vi "Display.vi"(8 "error in":errorcluster, 11 "Input (String) in":refnum<class "Gif - Input (String).lvclass">) -> (0 "error out":errorcluster, 3 "Input (String) out":refnum<class "Gif - Input (String).lvclass">)   [LabVIEW 2020, in "Pop-Up.lvlib" / "Gif - Input (String).lvclass"]
doc: "This vi will display the input pop up waiting for a type string input from the user while displaying a custom graphic to the user.\n\n<b>Code Developed By:</b>\nDaniel Coons\nTechnology Service Corporation\n1983 S Liberty Drive\nBloomington, IN 47403\nPhone: 812 558-7100\ndaniel.coons@tsc.com\nwww.tsc.com/atcs"
uses:
  Gif - Input (String).lvclass
  C:/Development/tsc-pop-up/Popup/Popup.lvclass
  C:/Development/tsc-pop-up/Gif/Gif Parent.lvclass
  Gif - Input (String).lvclass/Gif - Input (String).ctl
  Popup/Popup.lvclass/Popup.ctl
  Gif Parent.lvclass/Gif Parent.ctl
  Popup/Data Member Access/Read Theme.vi
  Read Delays.vi
  Read Gif Images.vi
  Theme/Theme.lvclass
  Popup/Popup.lvclass
  user32.dll
panel:
  in  "closer":bool
  out "header":bool
  in  "OK":bool
  in  "Input":string
  out "Input value out":string
  out "2D Picture":picture
  out "Message":string
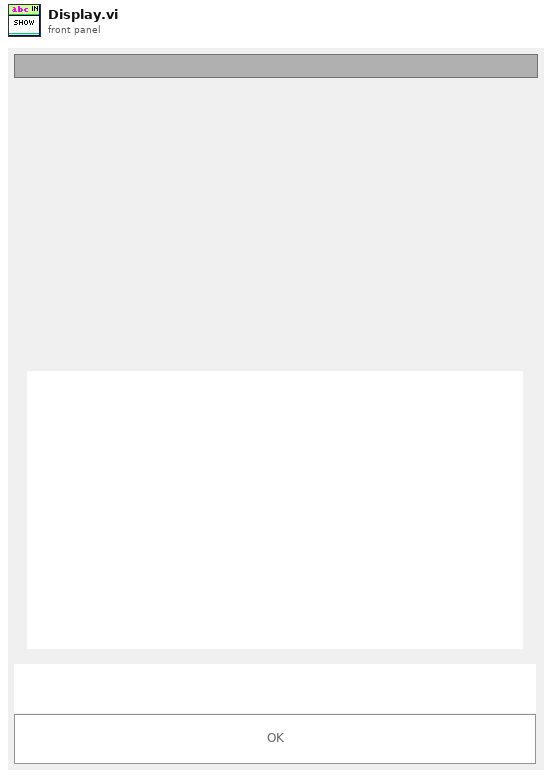
[diagram p1: front panel]
types:
  T1 = typedef "LVPoint32TypeDef.ctl" = cluster{"Horizontal":i32, "Vertical":i32}
  T2 = typedef "LVPositionTypeDef.ctl" = cluster{"Left":i32, "Top":i32}
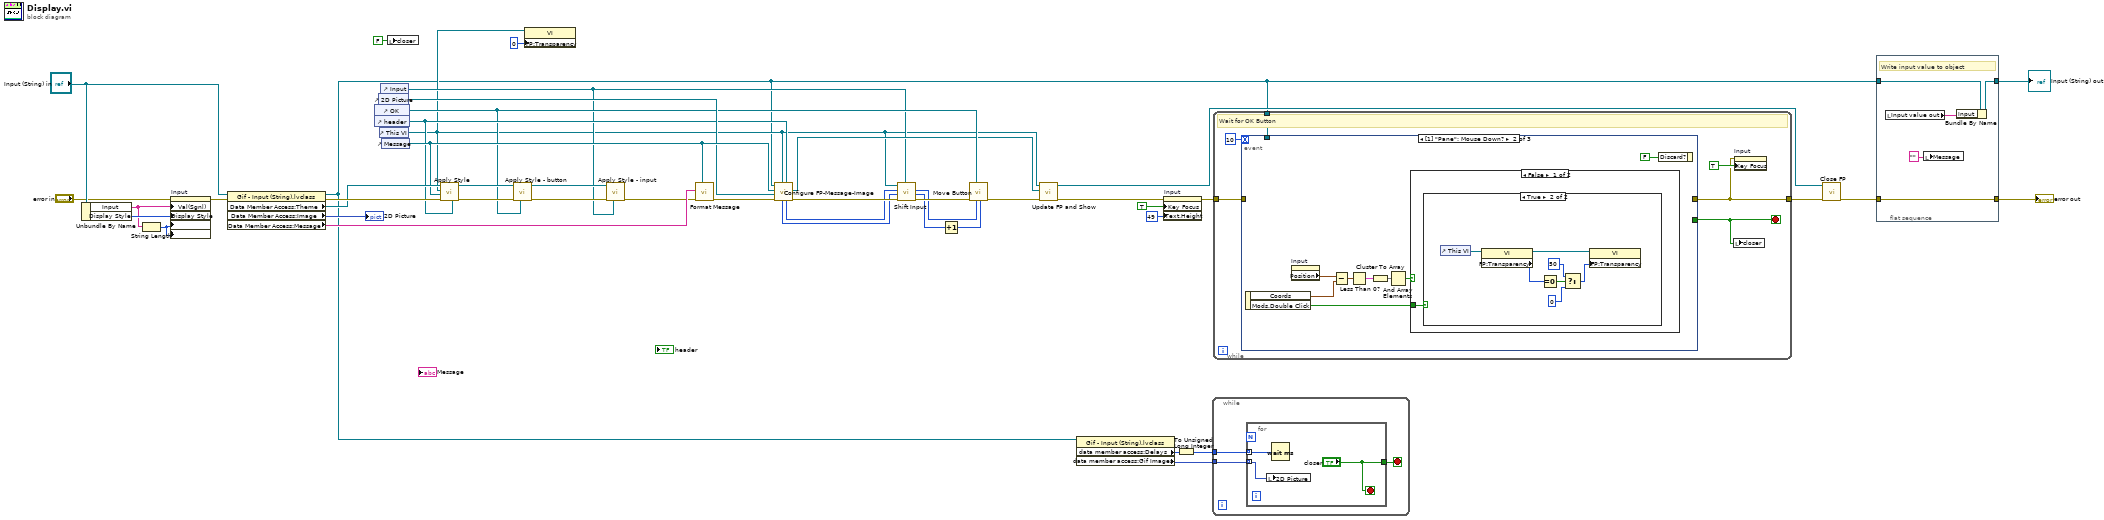
[diagram p0: block diagram]
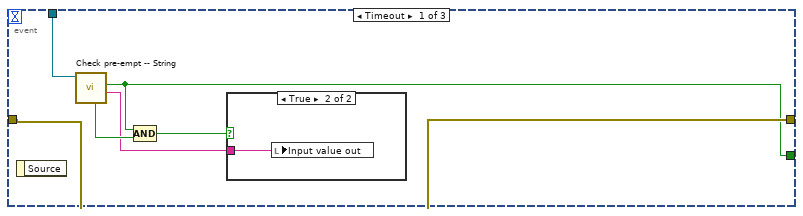
[diagram p2: hidden frame]
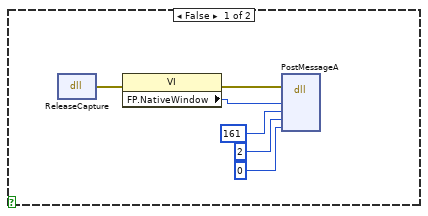
[diagram p4: hidden frame]
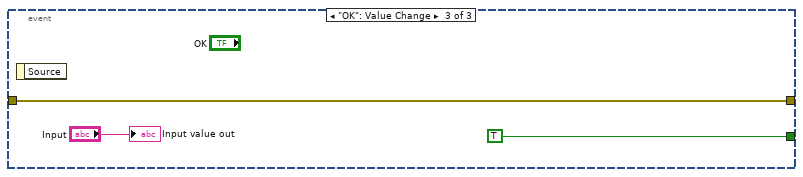
[diagram p6: hidden frame]
diagram:
  n1 = Unbundle By Name("Input (String) in") -> ("Input"=w12:string, "Display Style"=w13:u32)
  n2 = String Length(string=w12) -> (length=w11:i32)
  n3 = property on="Input" class="Str"(error in="error in", "Val(Sgnl)"=w12, "Display Style"=w13, "Text.Selection End"=w11, "Text.Selection Start"=w11) -> (error out=w42:errorcluster)  [unwired: 1 in, 1 out]
  n4 = property class="Gif - Input (String).lvclass"(reference="Input (String) in", error in=w42) -> (reference out=w2:refnum<class "Gif - Input (String).lvclass">, error out=w41:errorcluster, "Data Member Access:Theme"=w31:refnum<class "Theme.lvclass">, "Data Member Access:Image"=→"2D Picture":picture, "Data Member Access:Message"=w33:string)
  n5 = control-ref of="OK"() -> (w18:refnum<vi>)
  n6 = control-ref of="header"() -> (w24:refnum<vi>)
  n7 = control-ref of="2D Picture"() -> (w25:refnum<vi>)
  n8 = control-ref of="This VI"() -> (w6:refnum<vi>)
  n9 = control-ref of="Input"() -> (w10:refnum<vi>)
  n10 = control-ref of="Message"() -> (w26:refnum<vi>)
  n11 = local write "closer"(FALSE ("closer")) -> ()
  n12 = call "Apply Style.vi"("header ref"=w24, "error in (no error)"=w41, "message ref"=w26, "pop up ref"=w6, "Theme in"=w31) -> ("error out"=w32:errorcluster, "Theme out"=w29:refnum<class "Theme.lvclass">)  [unwired: 5 in]
  n13 = call "Apply Style - button.vi"("button ref"=w18, "error in (no error)"=w32, "Theme in"=w29) -> ("error out"=w30:errorcluster, "Theme out"=w27:refnum<class "Theme.lvclass">)  [unwired: 7 in]
  n14 = property on="Property Node" class="VI"(reference=w6, "FP:Transparency"=u8 0 ("Front Panel Window:Transparency")) -> ()  [unwired: 1 in, 2 out]
  n15 = call "Apply Style - input.vi"("input ref"=w10, "error in (no error)"=w30, "Theme in"=w27) -> ("error out"=w28:errorcluster)  [unwired: 7 in, 1 out]
  n16 = call "Format Message.vi"("formatted string"=w26, "error in"=w28, "String Input"=w33) -> ("error out"=w34:errorcluster)  [unwired: 7 in, 1 out]
  n17 = call "Configure FP-Message-Image.vi"("header ref"=w24, "Pop Up ref"=w6, "error in (no error)"=w34, "Image ref"=w25, "Message ref"=w26, "Popup in"=w2) -> ("error out"=w23:errorcluster, "Panel Ref"=w16:refnum<vi>, "Panel Width"=w21:i32, "Panel Height"=w20:i32)  [unwired: 1 in, 1 out]
  n18 = call "Shift Input.vi"("Control"=w10, "Error In"=w23, "Panel Height"=w20, "Panel Width"=w21, "Pop Up ref"=w6) -> ("Error Out"=w22:errorcluster, "Panel Height out"=w15:i32, "Panel Width out"=w17:i32)  [unwired: 4 in]
  n19 = Increment(x=w15) -> (x+1=w14:i32)
  n20 = call "Move Button.vi"("Panel Height"=w14, "Panel Width"=w17, "Button"=w18, "Error In"=w22) -> ("Error Out"=w19:errorcluster)  [unwired: 6 in, 1 out]
  n21 = call "Update FP and Show.vi"("error in (no error)"=w19, "Panel Ref"=w16, "VI in"=w6) -> ("error out"=w38:errorcluster, "VI out"=w8:refnum<vi>)  [unwired: 7 in]
  n22 = property class="Gif - Input (String).lvclass"(reference=w2) -> ("data member access:Delays"=w5:i32[], "data member access:Gif Images"=w4:picture[])  [unwired: 1 in, 2 out]
  n23 = property on="Input" class="Str"(error in=w38, "Key Focus"=TRUE, "Text.Height"=u32 49 ("Text.Size:Height")) -> (error out=w37:errorcluster)  [unwired: 1 in, 1 out]
  n24 = To Unsigned Long Integer(number=w5) -> (unsigned 32bit integer=w3:u32[])
  n25 = while {
    tunnel: w3 -> [w48]
    tunnel: w4 -> [w47]
    stop <- w49 stop-if-true
    n26 = for {
      tunnel: ["closer"] -> w49
      tunnel: w48 -> [w51] mode=indexing
      tunnel: w47 -> [w50] mode=indexing
      stop <- "closer" stop-if-true
      n27 = local write "2D Picture"(w50) -> ()
      n28 = Wait (ms)(milliseconds to wait=w51) -> ()  [unwired: 1 out]
    }
  }
  n29 = while {
    tunnel: w37 -> [w58]
    tunnel: [w54] -> w40
    tunnel: w2 -> [w56]
    stop <- w53 stop-if-true
    # "Wait for OK Button"
    n30 = event shown="[1] \"Pane\": Mouse Down?" {
      selector: _ -> [_ _ _]
      dyn-events: _ -> [_ _ _]
      timeout: 10 -> [_ _ _]
      tunnel: w58 -> [w60 _ w90]
      tunnel: [w60 _ w90] -> w54
      tunnel: [w59 _ TRUE] -> w53
      tunnel: w56 -> [w61 _ _]
      event Timeout {
        n31 = event-data() -> ()  [unwired: 1 in, 1 out]
        n32 = call "Check pre-empt -- String.vi"("_Popup in"=w61) -> ("Value?"=w62:string, "Pre-empted?"=w59:bool, "Type Match?"=w64:bool)  [unwired: 7 in, 1 out]
        n33 = Compound Arithmetic op=AND(w59, w64) -> (w63:bool)
        n34 = case shown="True" w63 {
          tunnel: w62 -> [_ w65]
          frame False {
          }
          frame True {
            n35 = local write "Input value out"(w65) -> ()
          }
        }
      }
      event Mouse Down? {
        n36 = event-data() -> ("Coords"=w67:T1, "Mods.Double Click"=w66:bool)  [unwired: 1 in]
        n37 = property on="Input" class="Str"() -> ("Position"=w68:T2)  [unwired: 2 in, 2 out]
        n38 = Subtract(x=w68, y=w67) -> (x-y=w69:T2)
        n39 = Less Than 0?(x=w69) -> (x < 0?=w70:cluster{"Left":bool, "Top":bool})
        n40 = Cluster To Array(cluster=w70) -> (array=w71:bool[])
        n41 = And Array Elements(Boolean array=w71) -> (logical AND=w72:bool)
        n42 = case shown="False" w72 {
          tunnel: w66 -> [w74 _]
          frame False {
            n43 = case shown="True" w74 {
              frame False {
                n44 = dll-call lib="user32.dll" fn="ReleaseCapture"() -> (error out=w78:errorcluster)  [unwired: 4 in, 1 out]
                n45 = property class="VI"(error in=w78) -> (error out=w79:errorcluster, "FP.NativeWindow"=w80:u64)  [unwired: 1 in, 1 out]
                n46 = dll-call lib="user32.dll" fn="PostMessageA"(error in=w79, "hWnd"=w80, "Msg"=161, "wParam"=2, "lParam"=0) -> ()  [unwired: 7 in, 2 out]
              }
              frame True {
                n47 = control-ref of="This VI"() -> (w87:refnum<vi>)
                n48 = property class="VI"(reference=w87) -> (reference out=w85:refnum<vi>, "FP:Transparency"=w86:u8)  [unwired: 1 in, 1 out]
                n49 = Equal To 0?(x=w86) -> (x = 0?=w84:bool)
                n50 = Select(t=u8 50, s=w84, f=u8 0) -> (s? t:f=w83:u8)
                n51 = property class="VI"(reference=w85, "FP:Transparency"=w83) -> ()  [unwired: 1 in, 2 out]
              }
            }
          }
          frame True {
          }
        }
        n52 = event-data("Discard?"=FALSE) -> ()  [unwired: 1 in, 1 out]
      }
      event "OK": Value Change {
        n53 = event-data() -> ()  [unwired: 1 in, 1 out]
        "Input value out" <- "Input"
      }
    }
    n54 = local write "closer"(w53) -> ()
    n55 = property on="Input" class="Str"(error in=w54, "Key Focus"=TRUE) -> ()  [unwired: 1 in, 2 out]
  }
  n56 = call "Close FP.vi"("error in (no error)"=w40, "VI in"=w8) -> ("error out"=w39:errorcluster)  [unwired: 9 in]
  n57 = flat-sequence {
    tunnel: w39 -> [w95]
    tunnel: [w95] -> w43
    tunnel: w2 -> [w94]
    tunnel: [w93] -> w44
    frame #0 {
      # "Write input value to object"
      n58 = local read "Input value out"() -> (w92:string)
      n59 = local write "Message"("" ("Message")) -> ()
      n60 = Bundle By Name(cluster=w94, "Input"=w92) -> (w93:refnum<class "Gif - Input (String).lvclass">)
    }
  }
  "error out" <- w43
  "Input (String) out" <- w44
